vi "Read Rank.vi"(8 "error in (no error)":errorcluster, 11 "Vector Path Group in":refnum<class "Vector 18GHz Path Group.lvclass">) -> (0 "error out":errorcluster, 2 "Rank":dbl, 3 "Vector Path Group out":refnum<class "Vector 18GHz Path Group.lvclass">)   [LabVIEW 2023, in "RFFixtureCharact.RFPM.lvlib" / "Vector 18GHz Path Group.lvclass"]
uses:
  Vector 18GHz Path Group.lvclass
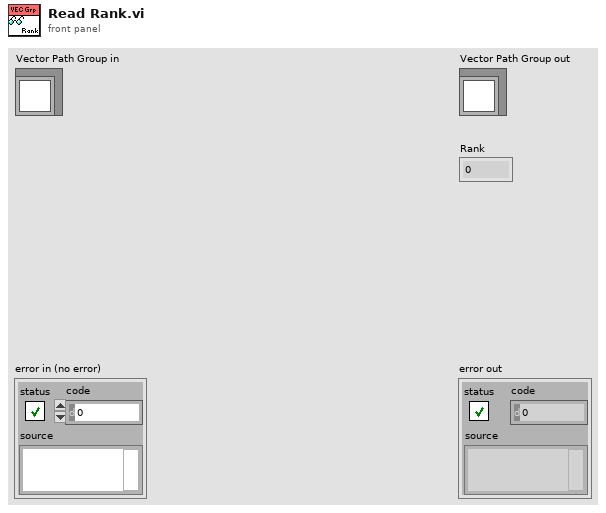
[diagram p1: front panel]
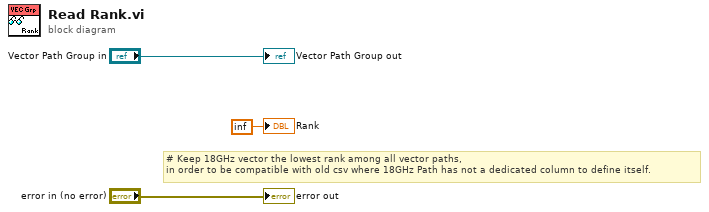
[diagram p0: block diagram]
diagram:
  # "# Keep 18GHz vector the lowest rank among all vector paths,\nin order to be compatible with old csv where 18GHz Path has not a dedicated column to define itself."
  "error out" <- "error in (no error)"
  "Vector Path Group out" <- "Vector Path Group in"
  "Rank" <- inf
